vi "Configure Active DUT Control Mode.vi"(8 "error in (no error)":errorcluster, 10 "Control Mode (Manual)":i32(ring) items=["Manual", "Automatic"], 11 "VISA resource name":refnum<visa-resource-name>) -> (0 "error out":errorcluster, 3 "VISA resource name out":refnum<visa-resource-name>)   [LabVIEW 2020, in "Rohde&Schwarz CMXP Base.lvlib"]
doc: "Selects the DUT control mode.\n\nAttribute:\nRSCMXPBASE_ATTR_ACTIVE_DUT_CONTROL_MODE\n\nRemote-control command:\n[CONFigure:]DUT:CONTrol:CMODe"
uses:
  <instrlib>/Rohde&Schwarz CMXP Base/Rohde&Schwarz CMXP Base.lvlib
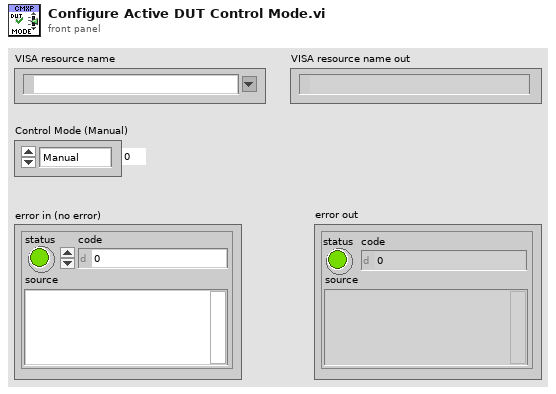
[diagram p1: front panel]
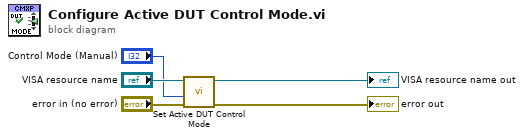
[diagram p0: block diagram]
diagram:
  n1 = call "Set Active DUT Control Mode"("error in (no error)"="error in (no error)", "Active DUT Control Mode (0 - Manual)"="Control Mode (Manual)", "instrument handle"="VISA resource name") -> ("error out"=→"error out":errorcluster, "instrument handle out"=→"VISA resource name out":refnum<visa-resource-name>)  [unwired: 7 in]
